vi "Osillioscope.vi"() -> ()   [LabVIEW 2025]
uses:
  <vilib>/Utility/error.llb/Trim Whitespace One-Sided.vi
  <vilib>/Instr/_visa.llb/VISA Configure Serial Port (Instr).vi
panel:
  in  "Trigger level":dbl
  in  "Trigger mode":enum16{"Auto", "Normal", ""}(ring)
  out "Boolean":bool
  in  "Vol/Div":dbl(knob) scale=0.0..1.0
  in  "Time/Div":dbl(knob) scale=1.0..1000.0
  in  "VISA resource name":refnum<visa-resource-name>
  in  "stop":bool
  out "Osillioscope":dbl(graph)
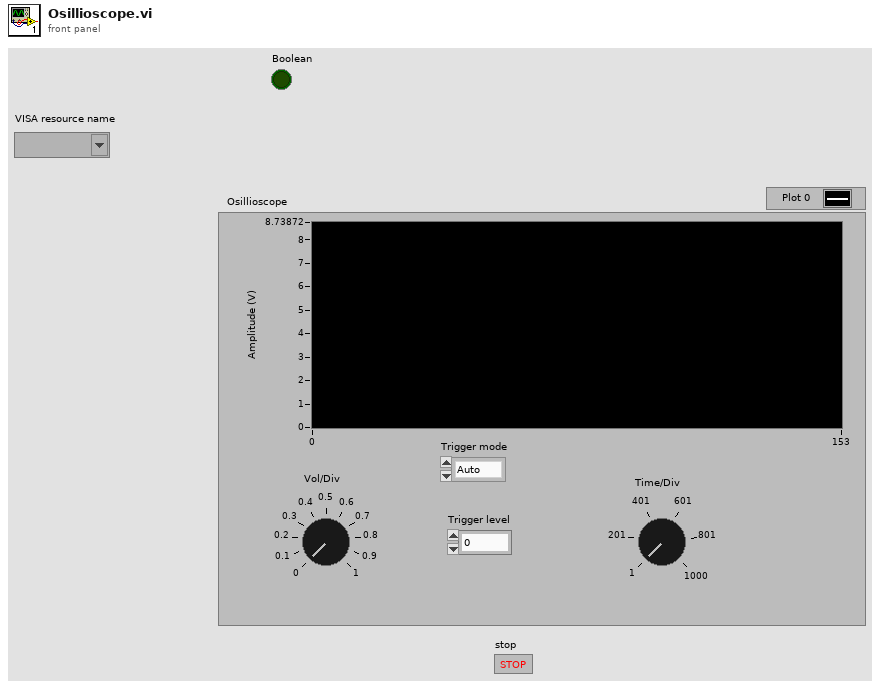
[diagram p1: front panel]
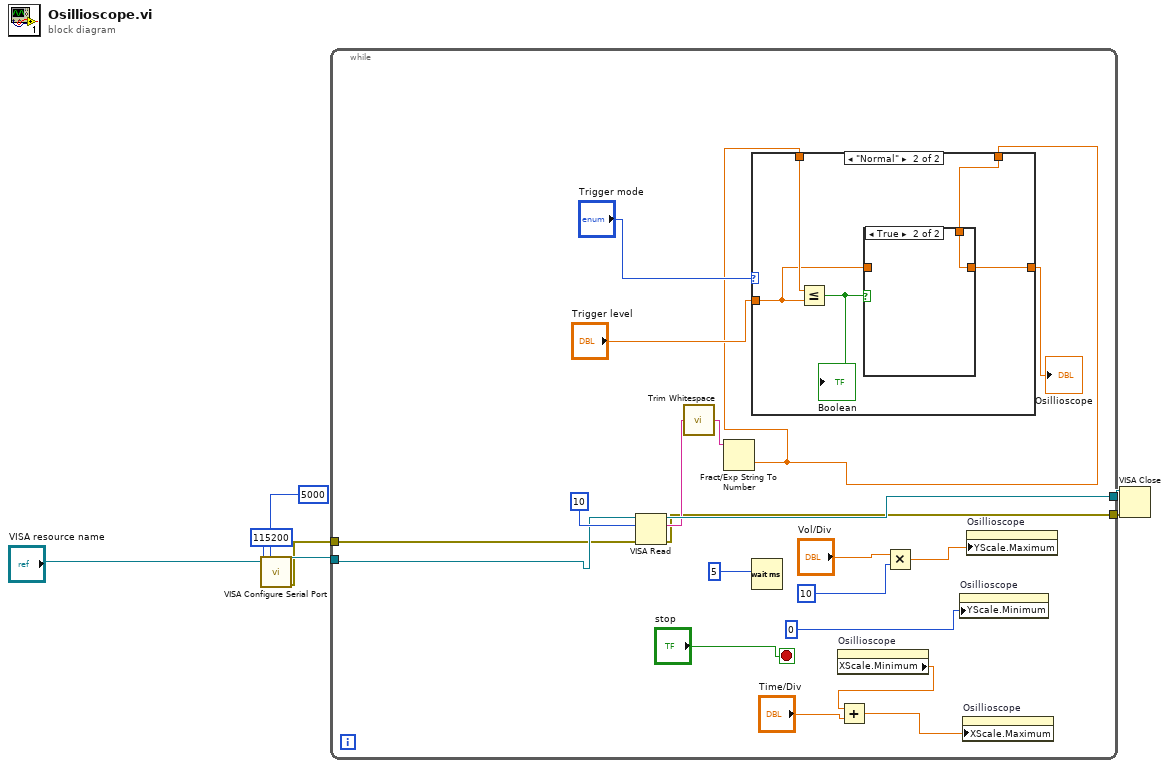
[diagram p0: block diagram]
diagram:
  n1 = call-poly "VISA Configure Serial Port"("VISA resource name"="VISA resource name", "timeout (10sec)"=u32 5000, "baud rate (9600)"=u32 115200) -> ("VISA resource name out"=w3:refnum<visa-resource-name>, "error out"=w1:errorcluster)  [unwired: 11 in]
  n2 = while {
    tunnel: w3 -> [w16]
    tunnel: [w26] -> w6
    tunnel: [w13] -> w2
    tunnel: w1 -> [w12]
    stop <- "stop" stop-if-true
    n3 = VISA Read(VISA resource name=w16, byte count=u32 10, error in (no error)=w12) -> (VISA resource name out=w26:refnum<visa-resource-name>, read buffer=w25:string, error out=w13:errorcluster)  [unwired: 1 out]
    n4 = call <vilib>:"Trim Whitespace.vi"("string"=w25) -> ("trimmed string"=w24:string)  [unwired: 1 in]
    n5 = Fract/Exp String To Number(string=w24) -> (number=w8:dbl)  [unwired: 3 in, 1 out]
    n6 = case shown="\"Normal\"" "Trigger mode" {
      tunnel: w8 -> [w28 w31]
      tunnel: [w28 w30] -> w9
      tunnel: w8 -> [_ w33]
      tunnel: "Trigger level" -> [_ w29]
      frame "Auto", Default {
      }
      frame "Normal" {
        n7 = Less Or Equal?(x=w33, y=w29) -> (x <= y?=w32:bool)
        "Boolean" <- w32
        n8 = case shown="True" w32 {
          tunnel: w31 -> [_ w35]
          tunnel: [w34 w35] -> w30
          tunnel: w29 -> [w34 _]
          frame False {
          }
          frame True {
          }
        }
      }
    }
    "Osillioscope" <- w9
    n9 = Wait (ms)(milliseconds to wait=u32 5 ("byte count")) -> ()  [unwired: 1 out]
    n10 = property on="Osillioscope" class="WFChart (strict)"() -> ("XScale.Minimum"=w14:dbl)  [unwired: 2 in, 2 out]
    n11 = Add(x=w14, y="Time/Div") -> (x+y=w17:dbl)
    n12 = Multiply(x="Vol/Div", y=10) -> (x*y=w20:dbl)
    n13 = property on="Osillioscope" class="WFChart (strict)"("YScale.Minimum"=0) -> ()  [unwired: 2 in, 2 out]
    n14 = property on="Osillioscope" class="WFChart (strict)"("XScale.Maximum"=w17) -> ()  [unwired: 2 in, 2 out]
    n15 = property on="Osillioscope" class="WFChart (strict)"("YScale.Maximum"=w20) -> ()  [unwired: 2 in, 2 out]
  }
  n16 = VISA Close(VISA resource name=w6, error in (no error)=w2) -> ()  [unwired: 1 out]
